vi "Motor_SetSpeed.vi"(8 "error in":errorcluster, 9 "Speed":dbl min=-1.0 max=1.0, 10 "PWM_Channel":T1=1 items=["Invalid"=0, "PWM1"=1, "PWM2"=2, "PWM9"=9, "PWM10"=10], 11 "FPGA_Ref_in":refnum<k20>) -> (0 "error out":errorcluster)   [LabVIEW 2009, in "Motor.lvlib"]
uses:
  Motor.lvlib
  PWM/PWM_Name.ctl
  ControllerType.ctl
  PWM.lvlib
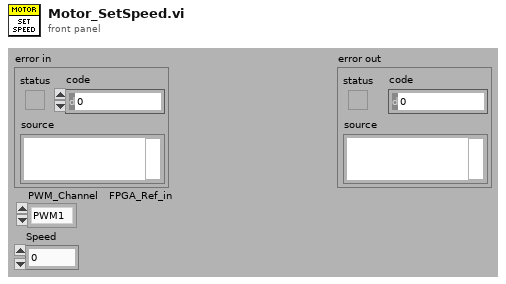
[diagram p1: front panel]
types:
  T1 = typedef "PWM.lvlib/PWM_Name.ctl" = u16
  T2 = typedef "Motor.lvlib/ControllerType.ctl" = u16
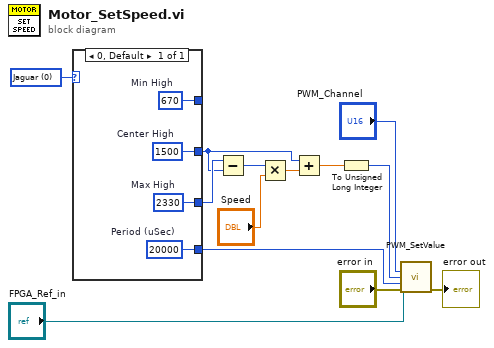
[diagram p0: block diagram]
diagram:
  w12 = T2 0 items=["Jaguar"] ("ControllerType")
  n1 = case shown="0, Default" w12 {
    tunnel: [w17] -> w5
    tunnel: [w16] -> _
    tunnel: [w15] -> w10
    tunnel: [w14] -> w11
    frame 0, Default {
      w14 = u32 2330  # Max High
      w15 = u32 1500  # Center High
      w16 = u32 670  # Min High
      w17 = u32 20000  # Period (uSec)
    }
  }
  n2 = Subtract(x=w11, y=w10) -> (x-y=w9:u32)
  n3 = Multiply(x=w9, y="Speed") -> (x*y=w7:dbl)
  n4 = Add(x=w10, y=w7) -> (x+y=w6:dbl)
  n5 = To Unsigned Long Integer(number=w6) -> (unsigned 32bit integer=w4:u32)
  n6 = call "PWM_SetValue.vi"("FPGA_Ref_in"="FPGA_Ref_in", "PWM"="PWM_Channel", "High (uSec)"=w4, "Period (uSec)"=w5, "error in"="error in") -> ("error out"=→"error out":errorcluster)  [unwired: 9 in, 1 out]
